vi "SDG50LoadArbitraryVolat.vi"(1 "WFM (Column) Number":i32, 2 "Array WFM":i16[](array[numeric]), 4 "Timeout (40000 ms)":u32=40000, 5 "WFM Source":u16(ring) items=["Single file", "Split files", "Array"], 6 "WFM Length":i32, 8 "error in (no error)":errorcluster, 9 "WFM Path":path=path "C:/Data/_SoftDevelopment/M8190/WFMs/WFMTst4.txt", 11 "VISA resource name":refnum<visa-resource-name>="USB0::0xF4EC::0x1101::SDG6XEBC5R0119::INSTR") -> (0 "error out":errorcluster, 3 "VISA resource name out":refnum<visa-resource-name>)   [LabVIEW 2018]
doc: "Creates and saves an arbitrary waveform in edit memory. \n\n<B>Note:</B>\n\nCreates an arbitrary waveform in edit memory and because of this, the waveform will remain stored on the instrument until deleted. If any sensitive information is contained in the arbitrary waveform, it is recommended that the waveform be deleted when finished."
uses:
  <vilib>/Utility/file.llb/Read From Spreadsheet File (I64).vi
panel:
  out "Attempts":i32
  # "Load waveform into arb\nmemory of a certain channel\nunder name 'ARB#'\nIf WFM alerady exists - use ClearArbitrary\n64M points in total per channel\nTimeout is not implemented, because this\nVI is inline-compatible, need external timeout\nincrease"
  # "No dots in the file name!"
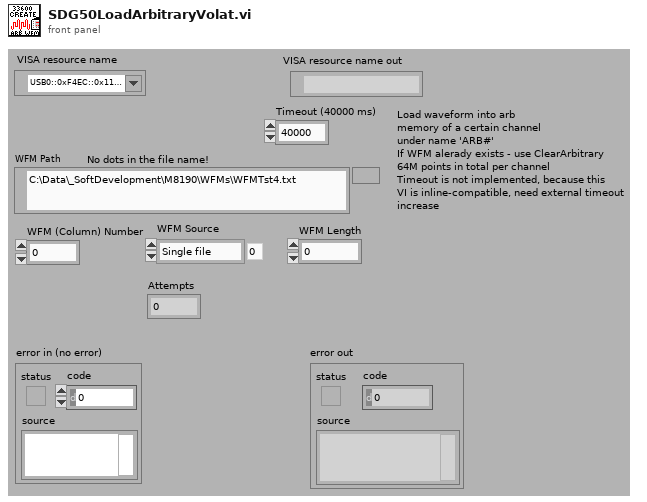
[diagram p1: front panel]
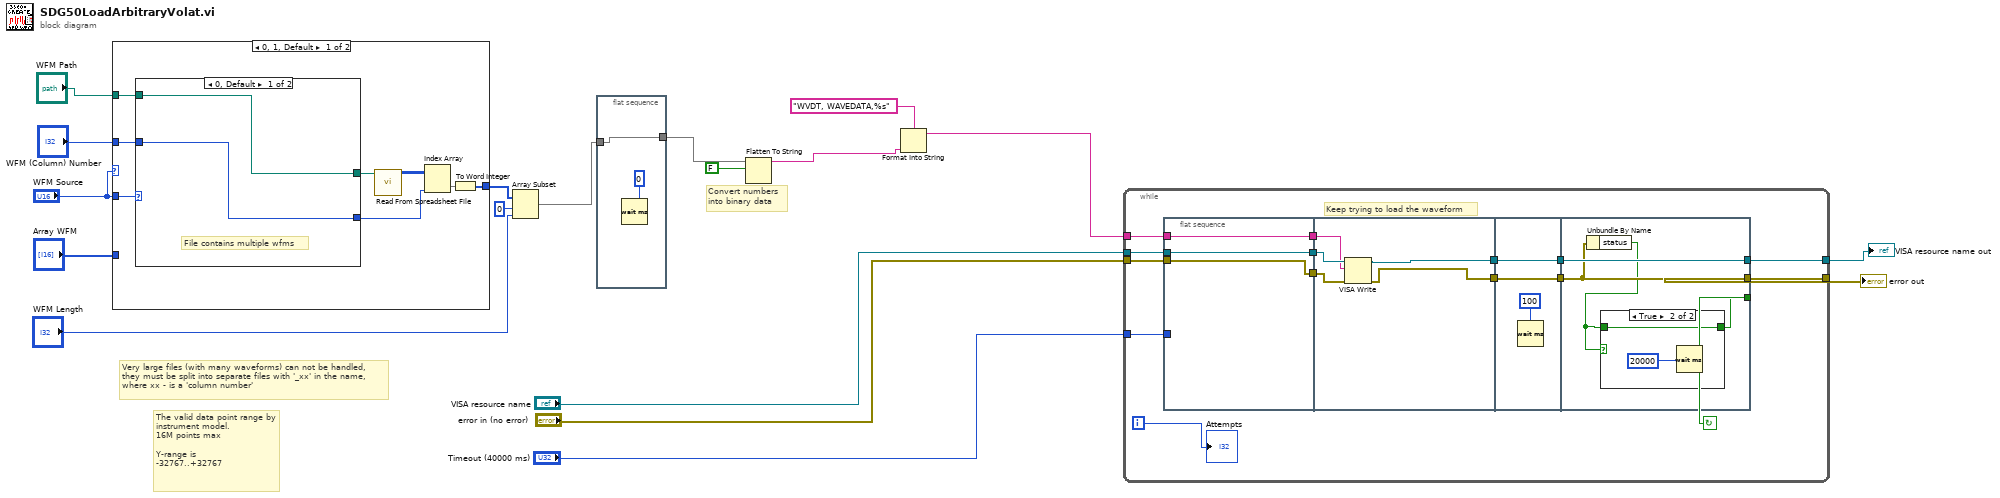
[diagram p0: block diagram]
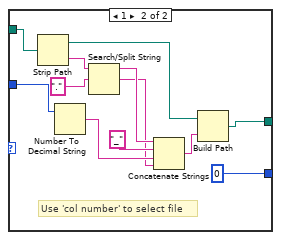
[diagram p2: hidden frame]
diagram:
  # "Very large files (with many waveforms) can not be handled,\nthey must be split into separate files with '_xx' in the name,\nwhere xx - is a 'column number'"
  # "Convert numbers\ninto binary data"
  # "The valid data point range by instrument model. \n16M points max\n\nY-range is\n-32767..+32767"
  n1 = case shown="0, 1, Default" "WFM Source" {
    tunnel: [w20 w41] -> w18
    tunnel: "WFM Path" -> [w25 _]
    tunnel: "WFM (Column) Number" -> [w24 _]
    tunnel: "WFM Source" -> [w21 _]
    tunnel: "Array WFM" -> [_ w41]
    frame 0, 1, Default {
      n2 = case shown="0, Default" w21 {
        tunnel: w25 -> [w28 w40]
        tunnel: w24 -> [w27 w37]
        tunnel: [w28 w31] -> w23
        tunnel: [w27 0 ("x")] -> w22
        frame 0, Default {
          # "File contains multiple wfms"
        }
        frame 1 {
          # "Use 'col number' to select file"
          n3 = Strip Path(path=w40) -> (stripped path=w32:path, name=w38:string)
          n4 = Number To Decimal String(number=w37) -> (decimal integer string=w34:string)  [unwired: 1 in]
          n5 = Search/Split String(string=w38, search string/char (-)=".") -> (substring before match=w36:string, match + rest of string=w33:string)  [unwired: 1 in, 1 out]
          n6 = Concatenate Strings(w36, "_", w34, w33) -> (w29:string)
          n7 = Build Path(base path=w32, name or relative path=w29) -> (appended path=w31:path)
        }
      }
      n8 = call-poly <vilib>:"Read From Spreadsheet File.vi"("file path (dialog if empty)"=w23) -> ("all rows"=w26:i64[][])  [unwired: 6 in, 4 out]
      n9 = Index Array(array=w26, index (col)=w22) -> (element=w19:i64[])  [unwired: 1 in]
      n10 = To Word Integer(number=w19) -> (16bit integer=w20:i16[])
    }
    frame 2 {
    }
  }
  n11 = Array Subset(array=w18, index=0 ("x"), length="WFM Length") -> (w2:i16[])
  n12 = flat-sequence {
    tunnel: w2 -> [w42]
    tunnel: [w42] -> w1
    frame #0 {
      n13 = Wait (ms)(milliseconds to wait=0 ("x")) -> ()  [unwired: 1 out]
    }
  }
  n14 = Flatten To String(anything=w1, prepend array or string size? (T)=FALSE) -> (data string=w3:string)  [unwired: 2 in, 2 out]
  n15 = Format Into String(format string="WVDT, WAVEDATA,%s", w3) -> (resulting string=w4:string)  [unwired: 2 in, 1 out]
  n16 = while {
    tunnel: w4 -> [w55]
    tunnel: "Timeout (40000 ms)" -> [w54]
    tunnel: "VISA resource name" -> [w53]
    tunnel: "error in (no error)" -> [w52]
    tunnel: [w51] -> w11
    tunnel: [w50] -> w10
    i -> [w44]
    stop <- w49 continue-if-true
    # "Keep trying to load the waveform"
    n17 = flat-sequence {
      tunnel: [w59] -> w58
      tunnel: [w60] -> w57
      tunnel: w55 -> [w61]
      tunnel: [w61] -> w56
      tunnel: w54 -> [_]
      tunnel: w53 -> [w59]
      tunnel: w52 -> [w60]
      tunnel: w58 -> [w65]
      tunnel: w57 -> [w66]
      tunnel: w56 -> [w64]
      tunnel: [w62] -> w48
      tunnel: [w63] -> w46
      tunnel: w48 -> [w69]
      tunnel: [w69] -> w47
      tunnel: w46 -> [w68]
      tunnel: [w68] -> w45
      tunnel: [w73] -> w50
      tunnel: [w72] -> w51
      tunnel: w47 -> [w72]
      tunnel: w45 -> [w73]
      tunnel: [w70] -> w49
      frame #0 {
      }
      frame #1 {
        n18 = VISA Write(VISA resource name=w65, write buffer=w64, error in (no error)=w66) -> (VISA resource name out=w63:refnum<visa-resource-name>, error out=w62:errorcluster)  [unwired: 1 out]
      }
      frame #2 {
        n19 = Wait (ms)(milliseconds to wait=100 ("x")) -> ()  [unwired: 1 out]
      }
      frame #3 {
        n20 = Unbundle By Name(w72) -> ("status"=w71:bool)
        n21 = case shown="True" w71 {
          tunnel: w71 -> [w74 w75]
          tunnel: [w74 w75] -> w70
          frame False {
          }
          frame True {
            n22 = Wait (ms)(milliseconds to wait=20000 ("x")) -> ()  [unwired: 1 out]
          }
        }
      }
    }
    "Attempts" <- w44
  }
  "error out" <- w11
  "VISA resource name out" <- w10
